vi "Introspection.vi"(8 "error in (no error)":errorcluster, 11 "CS++BaseActor in":refnum<class "CS++BaseActor.lvclass">) -> (0 "error out":errorcluster, 2 "CS++Messages":refnum<class "Message.lvclass">[](array[class]), 3 "CS++BaseActor out":refnum<class "CS++BaseActor.lvclass">)   [LabVIEW 2015, in "CS++BaseActor.lvlib" / "CS++BaseActor.lvclass"]
doc: "This vi delivers a list with all messages this actor reacts to. It executes a Core VI which has to be overwritten by each actor class."
uses:
  CS++BaseActor.lvclass
  <vilib>/ActorFramework/Message/Message.lvclass
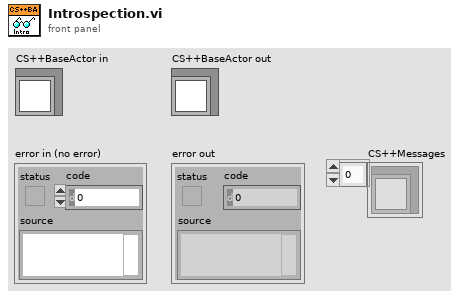
[diagram p1: front panel]
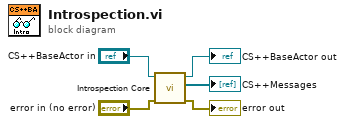
[diagram p0: block diagram]
diagram:
  n1 = call-dynamic "Introspection Core.vi"("error in (no error)"="error in (no error)", "CS++BaseActor in"="CS++BaseActor in") -> ("error out"=→"error out":errorcluster, "CS++Messages"=→"CS++Messages":refnum<class "Message.lvclass">[], "CS++BaseActor out"=→"CS++BaseActor out":refnum<class "CS++BaseActor.lvclass">)  [unwired: 7 in]
